vi "Get motion time.vi"(0 "Zaber":T1={"Serial port handle"="", "Axis"="", "Controller #"=0, "Min position"=0.0, "Max position"=0.0, "Min velocity"=0.0, "Max velocity"=0.0, "Firmware"="", "Device ID"=0, "Variable event"=refnum, "Variable ref"=refnum, "Resolution, usteps/step"=0, "Serial port semaphore"=refnum, "Joystick buttons"={"MinDir"=1, "MaxDir"=2, "MedSpeed"=5, "HighSpeed"=6}} {"Joystick buttons"."HighSpeed" min=1 max=25 step=1; "Joystick buttons"."MedSpeed" min=1 max=25 step=1; "Joystick buttons"."MaxDir" min=1 max=25 step=1; "Joystick buttons"."MinDir" min=1 max=25 step=1}, 2 "Distance, mm":dbl, 5 "error in":errorcluster) -> (14 "Zaber out":T1={"Serial port handle"="", "Axis"="", "Controller #"=0, "Min position"=0.0, "Max position"=0.0, "Min velocity"=0.0, "Max velocity"=0.0, "Firmware"="", "Device ID"=0, "Variable event"=refnum, "Variable ref"=refnum, "Resolution, usteps/step"=0, "Serial port semaphore"=refnum, "Joystick buttons"={"MinDir"=1, "MaxDir"=2, "MedSpeed"=5, "HighSpeed"=6}} {"Joystick buttons"."HighSpeed" min=1 max=25 step=1; "Joystick buttons"."MedSpeed" min=1 max=25 step=1; "Joystick buttons"."MaxDir" min=1 max=25 step=1; "Joystick buttons"."MinDir" min=1 max=25 step=1}, 16 "Motion time, s":dbl, 19 "error out":errorcluster)   [LabVIEW 2018]
uses:
  Zaber.ctl
  GenericDataEvent/GenericEvent.ctl
  ZaberVariables.ctl
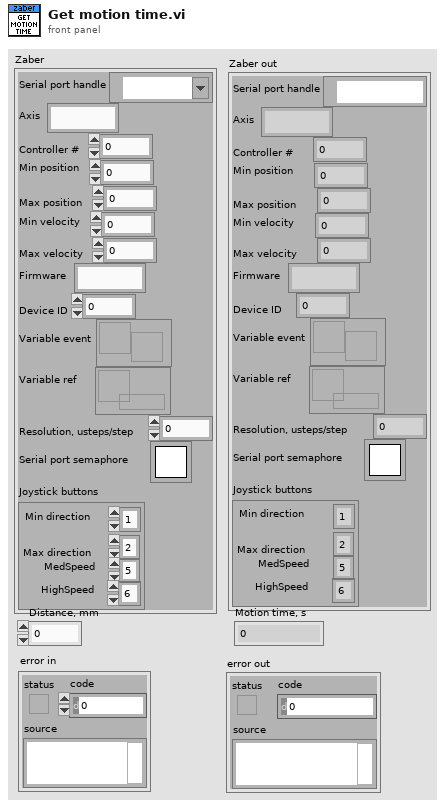
[diagram p1: front panel]
types:
  T1 = typedef "Zaber.ctl" = cluster{"Serial port handle":refnum<visa-resource-name>, "Axis":string, "Controller #":u8, "Min position":dbl, "Max position":dbl, "Min velocity":dbl, "Max velocity":dbl, "Firmware":string, "Device ID":i32, "Variable event":T2, "Variable ref":refnum<data-value>, "Resolution, usteps/step":i32, "Serial port semaphore":T3, "Joystick buttons":cluster{"MinDir":i32, "MaxDir":i32, "MedSpeed":i32, "HighSpeed":i32}}
  T2 = typedef "GenericEvent.ctl" = refnum<user-event>
  T3 = typedef "Semaphore RefNum" = refnum<k1>
  T4 = typedef "ZaberVariables.ctl" = cluster{"Position":i32, "Speed":i32, "Min soft position":dbl, "Max soft position":dbl, "Accelaration":i32}
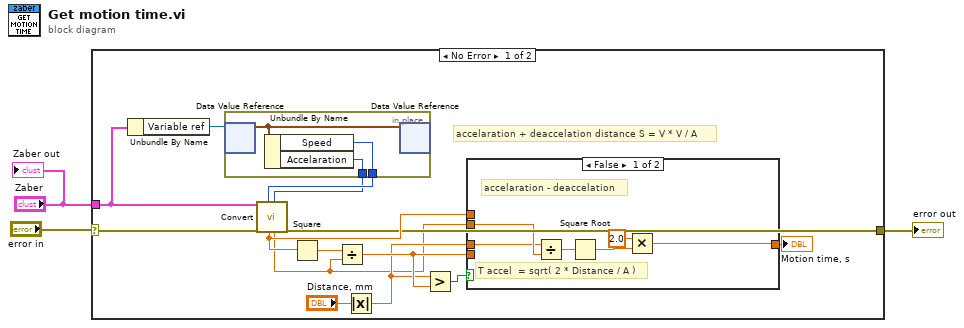
[diagram p0: block diagram]
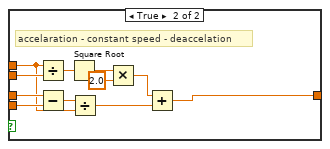
[diagram p2: hidden frame]
diagram:
  n1 = case shown="No Error" "error in" {
    selector: "error in" -> [w10 w38]
    tunnel: [w7 w38] -> w1
    tunnel: "Zaber" -> [w9 _]
    frame No Error {
      # "accelaration + deaccelation distance S = V * V / A"
      n2 = Unbundle By Name(w9) -> ("Variable ref"=w11:refnum<data-value>)
      n3 = in-place {
        in-place-border: [w19] -> w6
        in-place-border: [w18] -> w5
        n4 = in-place-dvr #1(w11) -> (w20:T4)  [unwired: 1 out]
        n5 = Unbundle By Name(w20) -> ("Speed"=w19:i32, "Accelaration"=w18:i32)
        n6 = in-place-dvr #1(w20) -> ()  [unwired: 2 out]
      }
      n7 = call "Convert.vi"("Zaber"=w9, "error in"=w10, "Velocity, counts"=w6, "Accelaration, counts"=w5) -> ("Velocity, mm/s"=w8:dbl, "Accelaration, mm/s/s"=w4:dbl, "error out"=w7:errorcluster)  [unwired: 7 in, 6 out]
      n8 = Square(x=w8) -> (x^2=w17:dbl)
      n9 = Divide(x=w17, y=w4) -> (x/y=w15:dbl)
      n10 = Absolute Value(x="Distance, mm") -> (abs(x)=w13:dbl)
      n11 = Greater?(x=w13, y=w15) -> (0:w16:bool)
      n12 = case shown="False" w16 {
        tunnel: w8 -> [_ w33]
        tunnel: w4 -> [w25 w37]
        tunnel: w13 -> [w21 w36]
        tunnel: w15 -> [_ w35]
        tunnel: [w22 w32] -> w12
        frame False {
          # "T accel  = sqrt( 2 * Distance / A )"
          # "accelaration - deaccelation"
          n13 = Divide(x=w21, y=w25) -> (x/y=w24:dbl)
          n14 = Square Root(x=w24) -> (sqrt(x)=w23:dbl)
          n15 = Multiply(x=2.0 ("y"), y=w23) -> (x*y=w22:dbl)
        }
        frame True {
          # "accelaration - constant speed - deaccelation"
          n16 = Divide(x=w33, y=w37) -> (x/y=w29:dbl)
          n17 = Subtract(x=w36, y=w35) -> (x-y=w34:dbl)
          n18 = Square Root(x=w29) -> (sqrt(x)=w28:dbl)
          n19 = Divide(x=w34, y=w33) -> (x/y=w30:dbl)
          n20 = Multiply(x=w28, y=2.0) -> (x*y=w27:dbl)
          n21 = Add(x=w27, y=w30) -> (x+y=w32:dbl)
        }
      }
      "Motion time, s" <- w12
    }
    frame Error {
    }
  }
  "error out" <- w1
  "Zaber out" <- "Zaber"
